vi "CLD 12 Sequencer State Machine.vi"() -> ()   [LabVIEW 2009]
doc: "CLD 12 exercise"
panel:
  out "Current Time Target":dbl
  in  "Stop Button":bool
  out "Time Elapsed":dbl
  out "Switch 3":bool
  out "Switch 2":bool
  out "Switch 1":bool
  in  "Start":bool
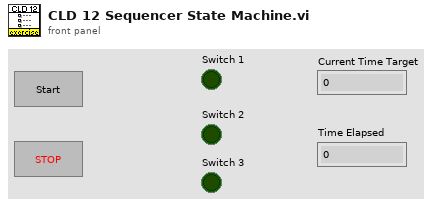
[diagram p1: front panel]
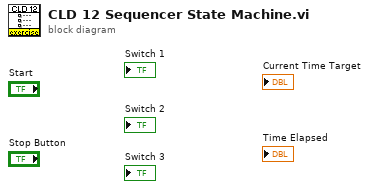
[diagram p0: block diagram]
diagram:
